vi "ProcessTraceTest.vi"() -> ()   [LabVIEW 2009]
panel:
  out "Waveform Chart":i32[][](graph)
  in  "Gain":i32=50000
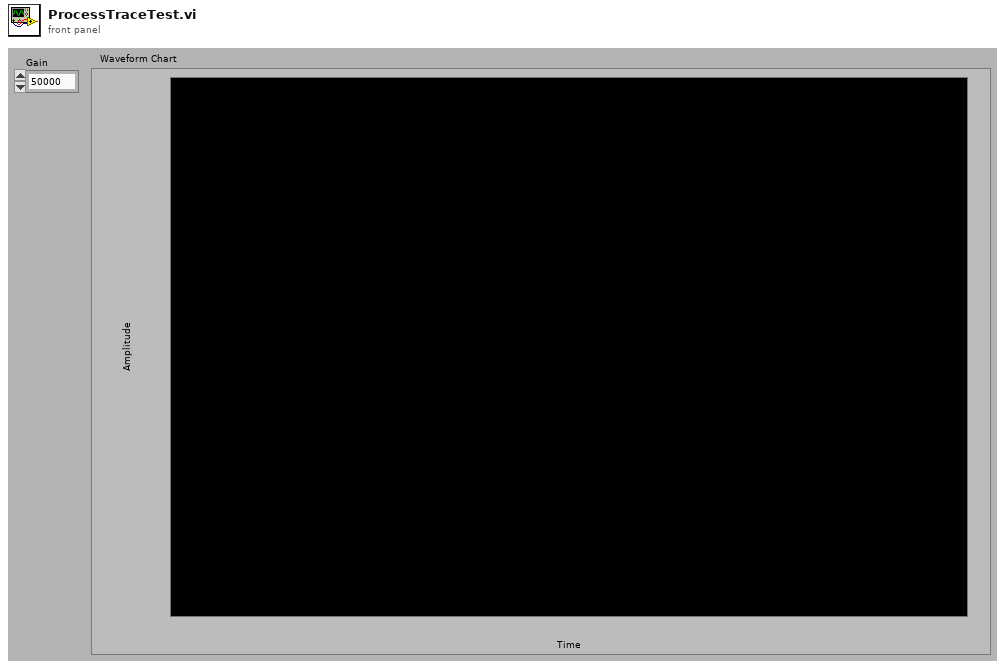
[diagram p1: front panel]
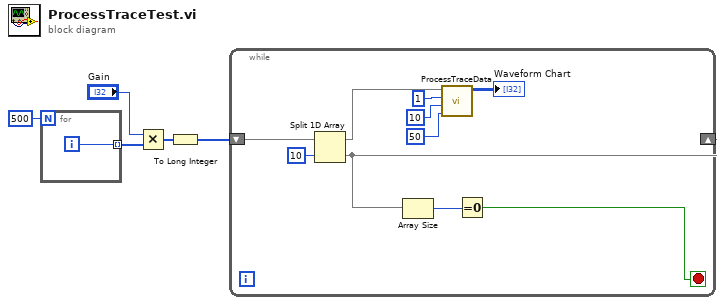
[diagram p0: block diagram]
diagram:
  n1 = for {
    N: 500 -> [_]
    tunnel: [w6] -> w3 mode=indexing
    i -> [w6]
  }
  n2 = Multiply(x="Gain", y=w3) -> (x*y=w5:i32[])
  n3 = To Long Integer(number=w5) -> (32bit integer=w1:i32[])
  n4 = while {
    shift-right: [w14] -> _
    shift-left: w1 -> [w16]
    stop <- w12 stop-if-true
    n5 = Split 1D Array(array=w16, index=10) -> (first subarray=w11:i32[], second subarray=w14:i32[])
    n6 = Array Size(array=w14) -> (size(s)=w13:i32)
    n7 = call "ProcessTraceData.vi"("Space"=50, "NumPoints"=10, "NumChans"=1, "Data"=w11) -> ("Waveform"=→"Waveform Chart":i32[][])  [unwired: 7 in]
    n8 = Equal To 0?(x=w13) -> (x = 0?=w12:bool)
  }
